vi "filas.vi"() -> ()   [LabVIEW 2016]
panel:
  out "# elements in queue":i32(slide) scale=0.0..1000.0
  in  "espera 2":u32
  out "indice 2":i32
  out "Waveform Chart 2":dbl(graph)
  out "Waveform Chart":dbl(graph)
  out "indice 1":i32
  in  "espera 1":u32
  in  "B1":bool
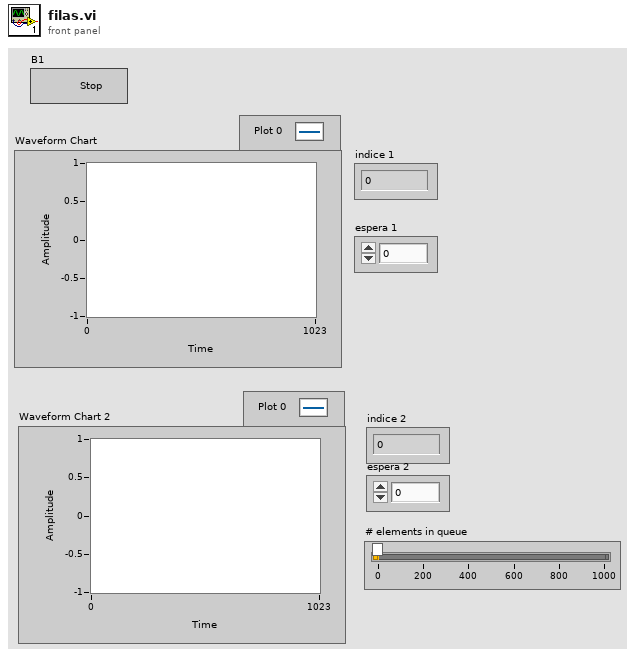
[diagram p1: front panel]
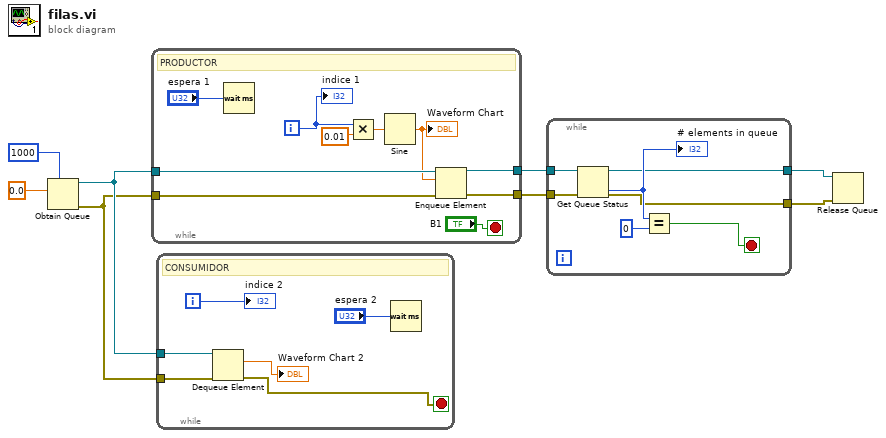
[diagram p0: block diagram]
diagram:
  n1 = Obtain Queue(max queue size (-1, unlimited)=1000, element data type=0.0) -> (queue out=w6:refnum<queue>, error out=w5:errorcluster)  [unwired: 3 in, 1 out]
  n2 = while {
    tunnel: w6 -> [w13]
    tunnel: w5 -> [w12]
    tunnel: [w10] -> w4
    tunnel: [w9] -> w3
    i -> [w16]
    stop <- "B1" stop-if-true
    # "PRODUCTOR"
    n3 = Wait (ms)(milliseconds to wait="espera 1") -> ()  [unwired: 1 out]
    n4 = Multiply(x=w16, y=0.01) -> (x*y=w15:dbl)
    n5 = Sine(x=w15) -> (sin(x)=w11:dbl)
    "Waveform Chart" <- w11
    n6 = Enqueue Element(queue=w13, element=w11, error in (no error)=w12) -> (queue out=w10:refnum<queue>, error out=w9:errorcluster)  [unwired: 1 in, 1 out]
    "indice 1" <- w16
  }
  n7 = while {
    tunnel: w5 -> [w22]
    tunnel: w6 -> [w21]
    i -> [w23]
    stop <- w19 stop-if-true
    # "CONSUMIDOR"
    n8 = Dequeue Element(queue=w21, error in (no error)=w22) -> (element=→"Waveform Chart 2":dbl, error out=w19:errorcluster)  [unwired: 1 in, 2 out]
    n9 = Wait (ms)(milliseconds to wait="espera 2") -> ()  [unwired: 1 out]
    "indice 2" <- w23
  }
  n10 = while {
    tunnel: w4 -> [w31]
    tunnel: w3 -> [w30]
    tunnel: [w26] -> w2
    tunnel: [w25] -> w1
    stop <- w27 stop-if-true
    n11 = Get Queue Status(queue=w31, error in (no error)=w30) -> (queue out=w26:refnum<queue>, error out=w25:errorcluster, # elements in queue=w29:i32)  [unwired: 1 in, 5 out]
    "# elements in queue" <- w29
    n12 = Equal?(x=w29, y=0) -> (x = y?=w27:bool)
  }
  n13 = Release Queue(queue=w2, error in (no error)=w1) -> ()  [unwired: 1 in, 3 out]
